vi "KepcoDCPwr Voltage List Example.vi"(0 "VISA resource name":refnum<visa-resource-name>="GPIB0::6::INSTR", 5 "Open & close":bool=TRUE, 7 "Model In":string, 11 "error in (no error)":errorcluster) -> (15 "error out":errorcluster)   [LabVIEW 2013]
doc: "Creates ramp of equal sized steps in voltage mode, loading into unit list array.\nWill cause the list to be executed by power supply.\n\nWhen Executed from another vi, insure all connections are wired to this function. \n\nThe boolean should be wired to FALSE so that the open and close for the resource does nto occur. \nwhile not important when using GPIB, in serial and in Lan type connections insures proper operation."
panel:
  in  "Exit":bool
  in  "Start":bool
  out "Instrument Error":errorcluster
  in  "Current":dbl=0.37 format="%.2f"
  out "Voltage vs Time":cluster{dbl[], dbl[]}(graph)
  in  "Stop":bool
  in  "Disable @ End":bool
  in  "# of Cycles":i32=1
  in  "Step change":dbl=1.0 min=0.0001 step=1.0 format="%.2f"
  in  "Dwell (sec)":dbl=0.1 min=0.00094 max=0.034 step=0.0001 format="%.4f"
  in  "End (Volts)":dbl=10.0 format="%.2f"
  in  "Start (Volts)":dbl format="%.2f"
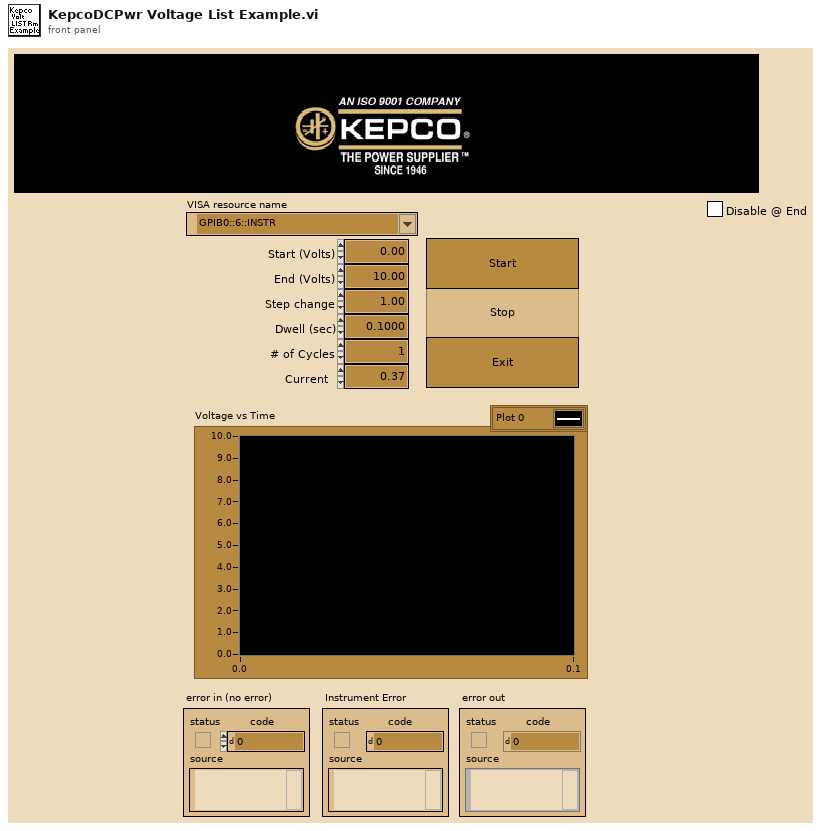
[diagram p1: front panel]
types:
  T1 = cluster{bool, "error code":i32, "error message":string}
  T2 = enum16{"Fixed", "List", "Transient", "External", "Gain", "Protect"}
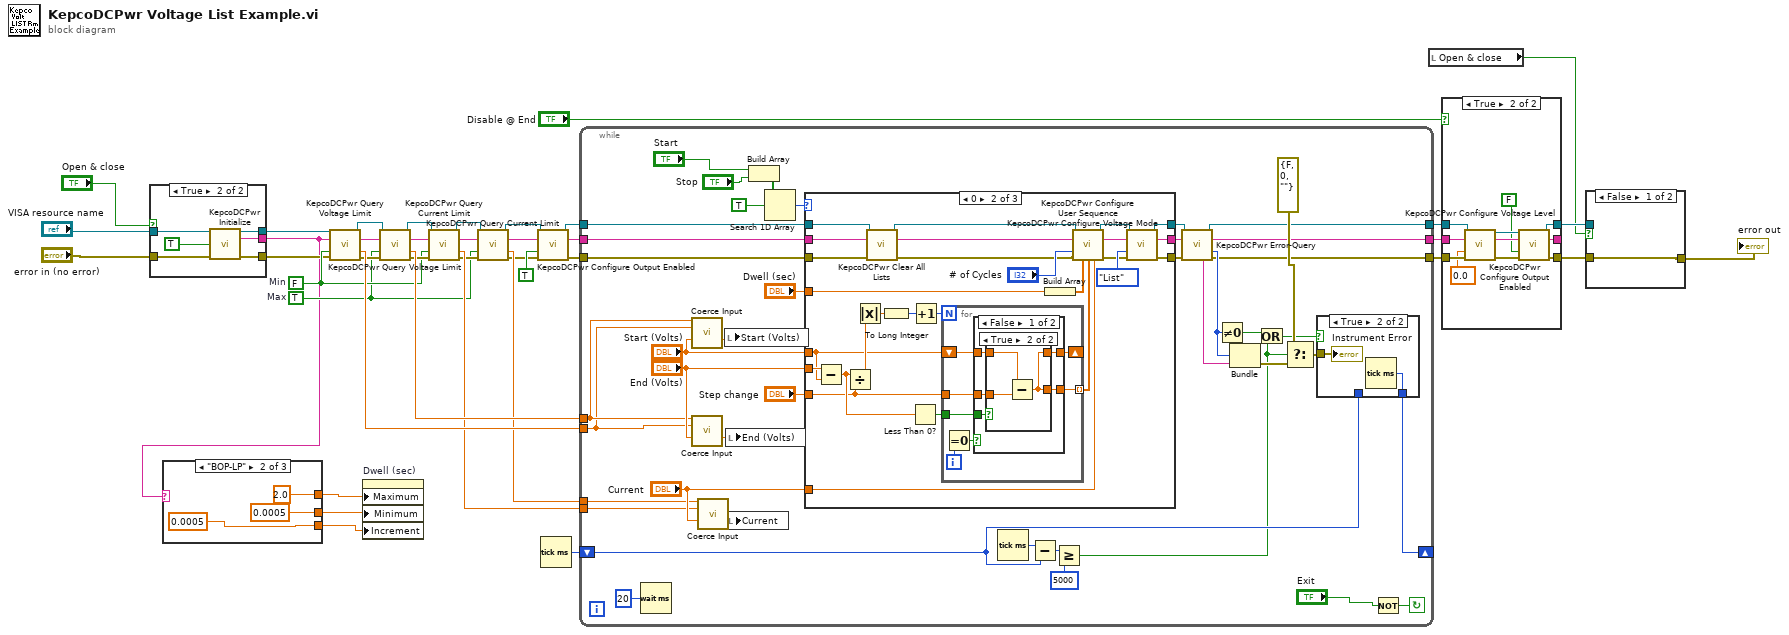
[diagram p0: block diagram]
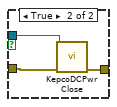
[diagram p2: hidden frame]
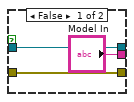
[diagram p3: hidden frame]
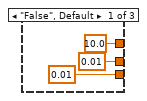
[diagram p4: hidden frame]
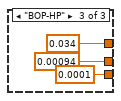
[diagram p5: hidden frame]
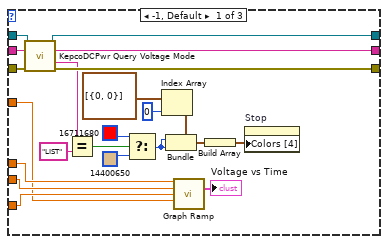
[diagram p7: hidden frame]
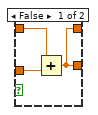
[diagram p8: hidden frame]
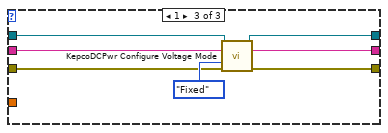
[diagram p10: hidden frame]
diagram:
  w17 = TRUE  # Max
  w18 = FALSE  # Min
  n1 = case shown="True" "Open & close" {
    tunnel: "error in (no error)" -> [w42 w48]
    tunnel: [w42 w47] -> w12
    tunnel: [w43 w46] -> w9
    tunnel: "VISA resource name" -> [w43 w45]
    tunnel: ["Model In" w44] -> w4
    frame False {
    }
    frame True {
      n2 = call "KepcoDCPwr Initialize.vi"("VISA Resource Name"=w45, "id query (True)"=TRUE, "error in (no error)"=w48) -> ("VISA Session Out"=w46:refnum<visa-resource-name>, "Model Out"=w44:string, "error out"=w47:errorcluster)  [unwired: 3 in, 7 out]
    }
  }
  n3 = case shown="\"BOP-LP\"" w4 {
    tunnel: [10.0 ("Data Entry Limits:Maximum") 2.0 ("Data Entry Limits:Maximum") 0.034 ("Data Entry Limits:Maximum")] -> w6
    tunnel: [0.01 ("Data Entry Limits:Minimum") 0.0005 ("Data Entry Limits:Minimum") 0.00094 ("Data Entry Limits:Minimum")] -> w5
    tunnel: [0.01 ("Data Entry Limits:Increment") 0.0005 ("Data Entry Limits:Increment") 0.0001 ("Data Entry Limits:Increment")] -> w3
    frame "False", Default {
    }
    frame "BOP-LP" {
    }
    frame "BOP-HP" {
    }
  }
  n4 = call "KepcoDCPwr Query Voltage Limit.vi"("VISA Session"=w9, "Model In"=w4, "Max Level (T),MIN LEVEL(F)"=w18, "error in (no error)"=w12) -> ("VISA Session Out"=w14:refnum<visa-resource-name>, "Model Out"=w23:string, "voltage level"=w30:dbl, "error out"=w24:errorcluster)  [unwired: 1 in, 7 out]
  n5 = property on="Dwell (sec)" class="DigNum (strict)"("Maximum"=w6, "Minimum"=w5, "Increment"=w3) -> ()  [unwired: 2 in, 2 out]
  n6 = call "KepcoDCPwr Query Voltage Limit.vi"("VISA Session"=w14, "Model In"=w23, "Max Level (T),MIN LEVEL(F)"=w17, "error in (no error)"=w24) -> ("VISA Session Out"=w15:refnum<visa-resource-name>, "Model Out"=w19:string, "voltage level"=w29:dbl, "error out"=w22:errorcluster)  [unwired: 1 in, 7 out]
  n7 = call "KepcoDCPwr Query Current Limit.vi"("VISA Session"=w15, "Model In"=w19, "Level"=w18, "error in (no error)"=w22) -> ("VISA Session Out"=w16:refnum<visa-resource-name>, "Model Out"=w20:string, "current limit"=w28:dbl, "error out"=w21:errorcluster)  [unwired: 1 in, 7 out]
  n8 = call "KepcoDCPwr Query Current Limit.vi"("VISA Session"=w16, "Model In"=w20, "Level"=w17, "error in (no error)"=w21) -> ("VISA Session Out"=w10:refnum<visa-resource-name>, "Model Out"=w11:string, "current limit"=w27:dbl, "error out"=w13:errorcluster)  [unwired: 1 in, 7 out]
  n9 = call "KepcoDCPwr Configure Output Enabled.vi"("VISA Session"=w10, "Model In"=w11, "Input enabled (True)"=TRUE, "error in (no error)"=w13) -> ("VISA Session Out"=w36:refnum<visa-resource-name>, "Model Out"=w35:string, "error out"=w34:errorcluster)  [unwired: 9 out]
  n10 = Tick Count (ms)() -> (millisecond timer value=w8:u32)
  n11 = while {
    shift-left: w8 -> [w63]
    shift-right: [w62] -> _
    tunnel: w27 -> [w87]
    tunnel: w28 -> [w88]
    tunnel: w29 -> [w82]
    tunnel: w30 -> [w81]
    tunnel: [w66] -> w31
    tunnel: [w64] -> w32
    tunnel: [w68] -> w33
    tunnel: w36 -> [w100]
    tunnel: w35 -> [w99]
    tunnel: w34 -> [w98]
    stop <- w97 continue-if-true
    n12 = Wait (ms)(milliseconds to wait=u32 20) -> ()  [unwired: 1 out]
    n13 = call "Coerce Input.vi"("Max"=w82, "Min"=w81, "Input"="Start (Volts)") -> ("Output"=w85:dbl)  [unwired: 12 out]
    n14 = call "Coerce Input.vi"("Max"=w82, "Min"=w81, "Input"="End (Volts)") -> ("Output"=w83:dbl)  [unwired: 12 out]
    n15 = call "Coerce Input.vi"("Max"=w87, "Min"=w88, "Input"="Current") -> ("Output"=w89:dbl)  [unwired: 12 out]
    n16 = local write "Start (Volts)"(w85) -> ()
    n17 = local write "End (Volts)"(w83) -> ()
    n18 = local write "Current"(w89) -> ()
    n19 = Build Array("Start", "Stop") -> (w94:bool[])
    n20 = Search 1D Array(1D array=w94, element=TRUE) -> (index of element=w93:i32)  [unwired: 1 in]
    n21 = case shown="0" w93 {
      tunnel: w100 -> [w120 w142 w173]
      tunnel: w99 -> [w118 w141 w175]
      tunnel: w98 -> [w116 w140 w177]
      tunnel: [w119 w136 w172] -> w69
      tunnel: [w117 w132 w174] -> w65
      tunnel: [w115 w131 w176] -> w67
      tunnel: "Step change" -> [w122 w130 _]
      tunnel: "End (Volts)" -> [w123 w129 _]
      tunnel: "Start (Volts)" -> [w124 w128 _]
      tunnel: "Dwell (sec)" -> [w121 w127 _]
      tunnel: "Current" -> [_ w126 _]
      frame -1, Default {
        n22 = call "KepcoDCPwr Query Voltage Mode.vi"("VISA Session"=w120, "Model In"=w118, "error in (no error)"=w116) -> ("VISA Session Out"=w119:refnum<visa-resource-name>, "Model Out"=w117:string, "Mode"=w111:string, "error out"=w115:errorcluster)  [unwired: 1 in, 8 out]
        n23 = Equal?(x=w111, y="LIST") -> (x = y?=w109:bool)
        n24 = Select(t=u32 16711680, s=w109, f=u32 14400650) -> (s? t:f=w106:u32)
        n25 = Index Array(array=cluster{u32, u32}[] [{0, 0}] ("Colors [4]"), index=0) -> (element=w113:cluster{u32, u32})
        n26 = Bundle(cluster=w113, w106, w106) -> (w112:cluster{u32, u32})
        n27 = call "Graph Ramp.vi"("Start (Volts)"=w124, "End (volts)"=w123, "Voltage Increment"=w122, "Dwell (sec)"=w121) -> ("Voltage vs Time"=→"Voltage vs Time":cluster{dbl[], dbl[]})  [unwired: 11 out]
        n28 = Build Array(w112) -> (w104:cluster{u32, u32}[])
        n29 = property on="Stop" class="Bool"("Colors [4]"=w104) -> ()  [unwired: 2 in, 2 out]
      }
      frame 0 {
        n30 = Subtract(x=w129, y=w128) -> (x-y=w149:dbl)
        n31 = Divide(x=w149, y=w130) -> (x/y=w146:dbl)
        n32 = Absolute Value(x=w146) -> (abs(x)=w147:dbl)
        n33 = call "KepcoDCPwr Clear All Lists.vi"("VISA Session"=w142, "Model In"=w141, "error in (no error)"=w140) -> ("VISA Session Out"=w143:refnum<visa-resource-name>, "Model Out"=w138:string, "error out"=w139:errorcluster)  [unwired: 1 in, 9 out]
        n34 = To Long Integer(number=w147) -> (32bit integer=w148:i32)
        n35 = Less Than 0?(x=w149) -> (x < 0?=w151:bool)
        n36 = Increment(x=w148) -> (x+1=w150:i32)
        n37 = for {
          N: w150 -> [_]
          tunnel: w151 -> [w159]
          tunnel: w130 -> [w157]
          shift-right: [w156] -> _
          shift-left: w128 -> [w158]
          tunnel: [w155] -> w145 mode=indexing
          i -> [w154]
          n38 = Equal To 0?(x=w154) -> (x = 0?=w153:bool)
          n39 = case shown="False" w153 {
            tunnel: w159 -> [w164 _]
            tunnel: w158 -> [w163 w171]
            tunnel: w157 -> [w162 _]
            tunnel: [w161 w171] -> w156
            tunnel: [w160 w171] -> w155
            frame False {
              n40 = case shown="True" w164 {
                tunnel: [w165 w168] -> w160
                tunnel: w163 -> [w167 w169]
                tunnel: w162 -> [w166 w170]
                tunnel: [w165 w168] -> w161
                frame False {
                  n41 = Add(x=w167, y=w166) -> (x+y=w165:dbl)
                }
                frame True {
                  n42 = Subtract(x=w169, y=w170) -> (x-y=w168:dbl)
                }
              }
            }
            frame True {
            }
          }
        }
        n43 = Build Array(w127) -> (w144:dbl[])
        n44 = call "KepcoDCPwr Configure User Sequence.vi"("VISA Session"=w143, "Model In"=w138, "# of Cycles"="# of Cycles", "error in (no error)"=w139, "Dwell (sec)"=w144, "List Data"=w145, "Limit Value"=w126) -> ("VISA Session Out"=w135:refnum<visa-resource-name>, "Model Out"=w133:string, "error out"=w134:errorcluster)  [unwired: 1 in, 5 out]
        n45 = call "KepcoDCPwr Configure Voltage Mode.vi"("VISA Session"=w135, "Model In"=w133, "Mode (Fixed)"=T2."List", "error in (no error)"=w134) -> ("VISA Session Out"=w136:refnum<visa-resource-name>, "Model Out"=w132:string, "error out"=w131:errorcluster)  [unwired: 2 in, 7 out]
      }
      frame 1 {
        n46 = call "KepcoDCPwr Configure Voltage Mode.vi"("VISA Session"=w173, "Model In"=w175, "Mode (Fixed)"=T2."Fixed", "error in (no error)"=w177) -> ("VISA Session Out"=w172:refnum<visa-resource-name>, "Model Out"=w174:string, "error out"=w176:errorcluster)  [unwired: 2 in, 7 out]
      }
    }
    n47 = Tick Count (ms)() -> (millisecond timer value=w79:u32)
    n48 = Subtract(x=w79, y=w63) -> (x-y=w78:u32)
    n49 = Greater Or Equal?(x=w78, y=u32 5000) -> (x >= y?=w61:bool)
    n50 = call "KepcoDCPwr Error-Query.vi"("VISA Session"=w69, "Model In"=w65, "error in (no error)"=w67) -> ("VISA Session Out"=w68:refnum<visa-resource-name>, "Model Out"=w64:string, "error code"=w72:i32, "error message"=w71:string, "error out"=w66:errorcluster)  [unwired: 1 in, 7 out]
    n51 = Not Equal To 0?(x=w72) -> (x != 0?=w73:bool)
    n52 = Bundle(w73, "error code"=w72, "error message"=w71) -> (w74:T1)  [unwired: 1 out]
    n53 = Or(x=w73, y=w61) -> (x .or. y?=w70:bool)
    n54 = Select(t=T1 {FALSE, "error code"=0, "error message"=""}, s=w61, f=w74) -> (s? t:f=w75:T1)
    n55 = case shown="True" w70 {
      tunnel: [w101 w103] -> w62
      tunnel: w63 -> [w101 _]
      tunnel: w75 -> [_ w102]
      frame False {
      }
      frame True {
        n56 = Tick Count (ms)() -> (millisecond timer value=w103:u32)
        "Instrument Error" <- w102
      }
    }
    n57 = Not(x="Exit") -> (.not. x?=w97:bool)
  }
  n58 = local read "Open & close"() -> (w1:bool)
  n59 = case shown="True" "Disable @ End" {
    tunnel: w33 -> [w181 w192]
    tunnel: w32 -> [w180 w191]
    tunnel: w31 -> [w179 w190]
    tunnel: [w179 w185] -> w39
    tunnel: [w181 w184] -> w40
    tunnel: [w180 w183] -> _
    frame False {
    }
    frame True {
      n60 = call "KepcoDCPwr Configure Voltage Level.vi"("VISA Session"=w192, "Model In"=w191, "level (0.0 volts)"=0.0, "error in (no error)"=w190) -> ("VISA Session Out"=w188:refnum<visa-resource-name>, "Model Out"=w187:string, "error out"=w186:errorcluster)  [unwired: 1 in, 8 out]
      n61 = call "KepcoDCPwr Configure Output Enabled.vi"("VISA Session"=w188, "Model In"=w187, "Input enabled (True)"=FALSE ("output enabled (True)"), "error in (no error)"=w186) -> ("VISA Session Out"=w184:refnum<visa-resource-name>, "Model Out"=w183:string, "error out"=w185:errorcluster)  [unwired: 9 out]
    }
  }
  n62 = case shown="False" w1 {
    tunnel: w40 -> [_ w196]
    tunnel: w39 -> [w193 w195]
    tunnel: [w193 w194] -> w37
    frame False {
    }
    frame True {
      n63 = call "KepcoDCPwr Close.vi"("VISA Session"=w196, "error in (no error)"=w195) -> ("error out"=w194:errorcluster)  [unwired: 13 out]
    }
  }
  "error out" <- w37
